vi "Get Backlog.vi"(8 "error in (no error)":errorcluster, 11 "IntanElectrophysiology in":refnum<class "IntanElectrophysiology.lvclass">) -> (0 "error out":errorcluster, 2 "Backlog":u32, 3 "IntanElectrophysiology out":refnum<class "IntanElectrophysiology.lvclass">)   [LabVIEW 2014, in "IntanElectrophysiology.lvclass"]
uses:
  IntanElectrophysiology.lvclass
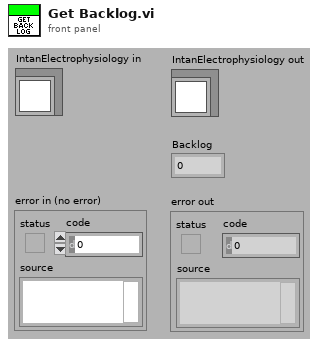
[diagram p1: front panel]
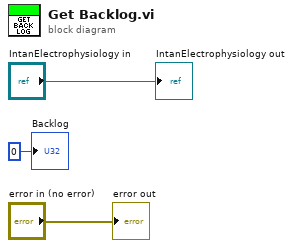
[diagram p0: block diagram]
diagram:
  "error out" <- "error in (no error)"
  "IntanElectrophysiology out" <- "IntanElectrophysiology in"
  "Backlog" <- u32 0 ("Backlog")
